vi "GOOPUtil_GetClassMembers.vi"(0 "LVClassPath":path, 5 "error in (no error)":errorcluster) -> (14 "MemberPaths":T1[](array[typedef]), 19 "error out":errorcluster)   [LabVIEW 2012, in "GOOPUtility.lvlib"]
doc: "Returns all class members paths, names and scopes (except the util VIs) from a given GOOP class path.\n\nNote: This will not work if the .lvclass file is inside an .exe file.\n\nThis is a collection of generic GOOP utility VIs. Please notice that it is important that the frontpanel of the Create, Destroy and GetObjectStatus is not removed when building an application."
uses:
  <vilib>/addons/GOOPUtility/GOOPUtility.lvlib
  <vilib>/addons/GOOPUtility/GOOPUtil_MemberDefinition.ctl
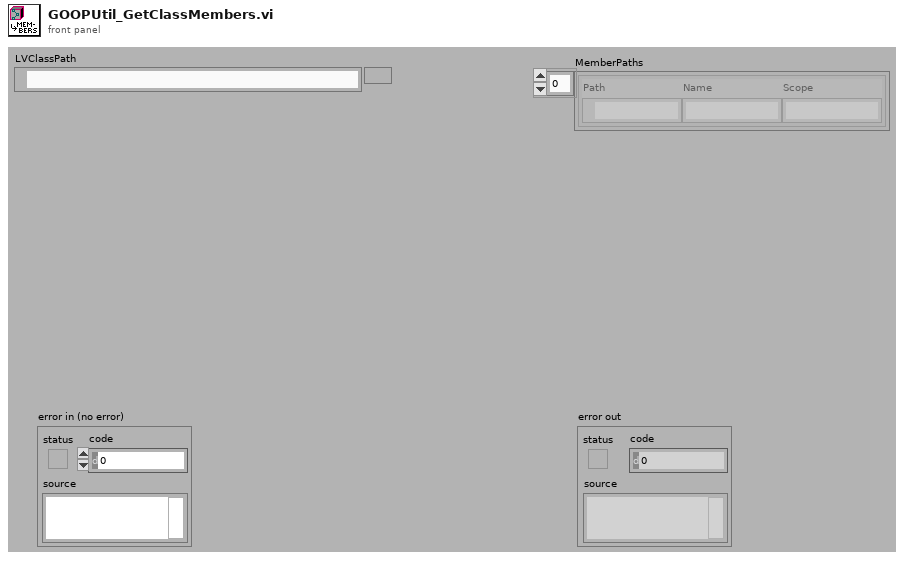
[diagram p1: front panel]
types:
  T1 = typedef "GOOPUtility.lvlib/GOOPUtil_MemberDefinition.ctl" = cluster{"Path":path, "Name":string, "Scope":string}
  T2 = enum16{"open", "replace", "create", "open or create", "replace or create", "replace or create with confirmation"}
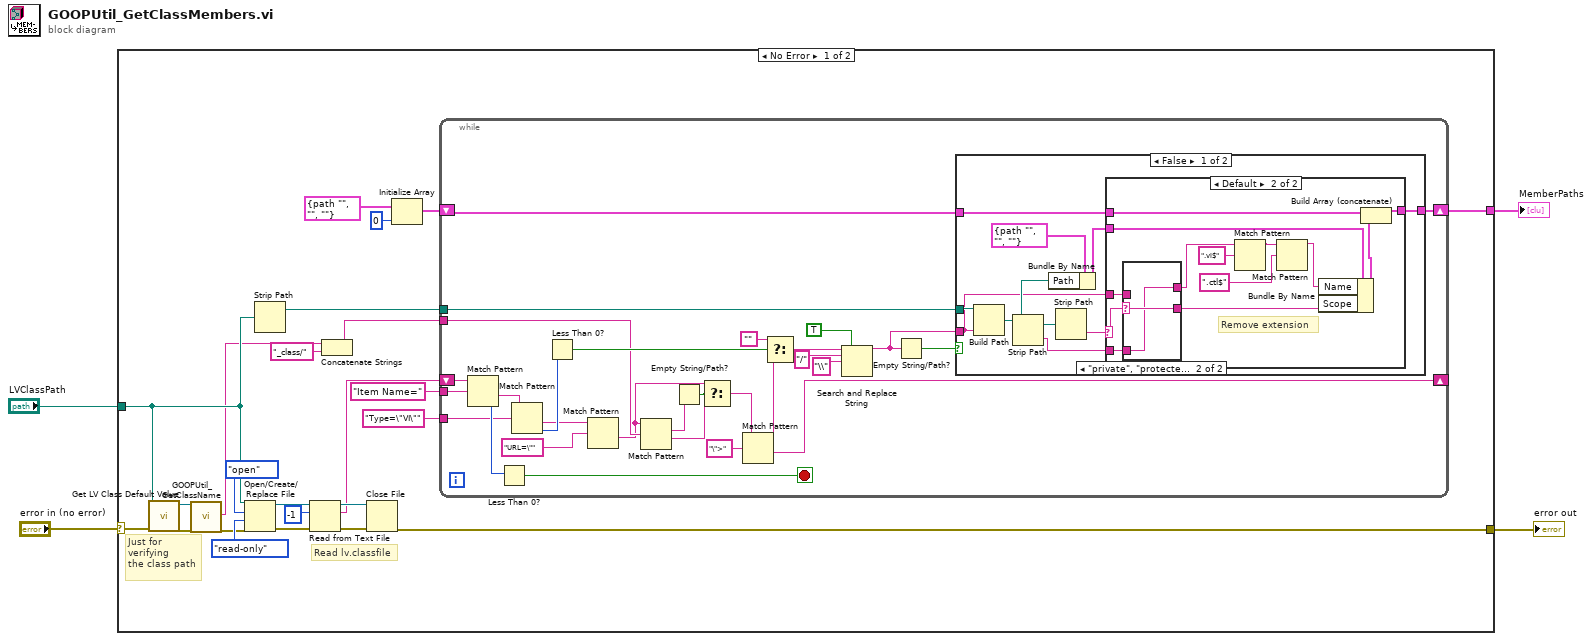
[diagram p0: block diagram]
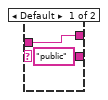
[diagram p3: hidden frame]
diagram:
  n1 = case shown="No Error" "error in (no error)" {
    selector: "error in (no error)" -> [w17 w87]
    tunnel: [w19 w87] -> w3
    tunnel: "LVClassPath" -> [w16 _]
    tunnel: [w14 _] -> w1
    frame No Error {
      # "Read lv.classfile"
      # "Just for\nverifying\nthe class path"
      n2 = call <vilib>:"Get LV Class Default Value.vi"("error in (no error)"=w17, "class path"=w16) -> ("error out"=w10:errorcluster, "object"=w9:refnum<class>)  [unwired: 8 in]
      n3 = call <vilib>:"GOOPUtil_GetClassName.vi"("LabVIEW Object"=w9, "error in (no error)"=w10) -> ("Class Name"=w7:string, "error out"=w8:errorcluster)  [unwired: 13 in, 3 out]
      n4 = Open/Create/Replace File(file path (use dialog)=w16, error in=w8, operation (0:open)=T2."open", access (0:read/write)=enum16{"read/write", "read-only", "write-only"}."read-only") -> (refnum out=w27:refnum<file>, error out=w26:errorcluster)  [unwired: 2 in, 1 out]
      n5 = Strip Path(path=w16) -> (stripped path=w15:path)  [unwired: 1 out]
      n6 = Read from Text File(file (use dialog)=w27, count=-1, error in=w26) -> (refnum out=w23:refnum<file>, text=w20:string, error out=w24:errorcluster)  [unwired: 2 out]
      n7 = Concatenate Strings(w7, "_class/" ("string")) -> (w5:string)
      n8 = Close File(refnum=w23, error in=w24) -> (error out=w19:errorcluster)  [unwired: 1 out]
      n9 = Initialize Array(T1 {"Path"=path "", "Name"="", "Scope"=""} ("Member"), 0 ("dimension size")) -> (w13:T1[])
      n10 = while {
        shift-right: [w44] -> _
        shift-left: w20 -> [w57]
        tunnel: "Item Name=" ("Search Tag") -> [w53]
        tunnel: "Type=\"VI\"" ("regular expression") -> [w52]
        shift-right: [w35] -> w14
        shift-left: w13 -> [w38]
        tunnel: w15 -> [w37]
        tunnel: w5 -> [w34]
        stop <- w54 stop-if-true
        n11 = Match Pattern(string=w57, regular expression=w53) -> (after substring=w56:string, offset past match=w55:i32)  [unwired: 3 out]
        n12 = Less Than 0?(x=w55) -> (x < 0?=w54:bool)
        n13 = Match Pattern(string=w56, regular expression=w52) -> (after substring=w48:string, offset past match=w51:i32)  [unwired: 3 out]
        n14 = Less Than 0?(x=w51) -> (x < 0?=w49:bool)
        n15 = Match Pattern(string=w48, regular expression="URL=\"" ("search string/char (-)")) -> (after substring=w31:string)  [unwired: 4 out]
        n16 = Match Pattern(string=w31, regular expression=w34) -> (match substring=w33:string, after substring=w30:string)  [unwired: 3 out]
        n17 = Empty String/Path?(string/path=w33) -> (empty?=w32:bool)
        n18 = Select(t=w31, s=w32, f=w30) -> (s? t:f=w29:string)
        n19 = Match Pattern(string=w29, regular expression="\">" ("search string/char (-)")) -> (before substring=w45:string, after substring=w44:string)  [unwired: 3 out]
        n20 = Select(t="", s=w49, f=w45) -> (s? t:f=w43:string)
        n21 = Search and Replace String(replace all?=TRUE ("replace all? (F)"), input string=w43, search string="/" ("search string/char (-)"), replace string="\\" ("search string/char (-)")) -> (result string=w36:string)  [unwired: 1 in, 6 out]
        n22 = Empty String/Path?(string/path=w36) -> (empty?=w39:bool)
        n23 = case shown="False" w39 {
          tunnel: w38 -> [w67 w86]
          tunnel: w37 -> [w66 _]
          tunnel: w36 -> [w59 _]
          tunnel: [w65 w86] -> w35
          frame False {
            n24 = Build Path(base path=w66, name or relative path=w59) -> (appended path=w61:path)
            n25 = Strip Path(path=w61) -> (stripped path=w64:path, name=w58:string)
            n26 = Bundle By Name(cluster=T1 {"Path"=path "", "Name"="", "Scope"=""} ("Member"), "Path"=w61) -> (w60:T1)
            n27 = Strip Path(path=w64) -> (name=w63:string)  [unwired: 1 out]
            n28 = case shown="Default" w63 {
              selector: w63 -> [_ w77]
              tunnel: w67 -> [w68 w81]
              tunnel: [w68 w78] -> w65
              tunnel: w60 -> [_ w80]
              tunnel: w59 -> [_ w75]
              tunnel: w58 -> [_ w74]
              frame "utils" {
                # "Don't include the utils VIs that is only for\nthe GOOP implementation."
              }
              frame Default {
                # "Remove extension"
                n29 = case shown="\"private\", \"protected\"" w77 {
                  selector: w77 -> [_ w85]
                  tunnel: ["public" w85] -> w76
                  tunnel: w75 -> [w82 _]
                  tunnel: w74 -> [_ w84]
                  tunnel: [w82 w84] -> w72
                  frame Default {
                  }
                  frame "private", "protected" {
                  }
                }
                n30 = Match Pattern(string=w72, regular expression=".vi$") -> (before substring=w71:string)  [unwired: 1 in, 3 out]
                n31 = Match Pattern(string=w71, regular expression=".ctl$") -> (before substring=w70:string)  [unwired: 1 in, 3 out]
                n32 = Bundle By Name(cluster=w80, "Name"=w70, "Scope"=w76) -> (w79:T1)
                n33 = Build Array (concatenate)(w81, w79) -> (w78:T1[])
              }
            }
          }
          frame True {
            # "False alarm..."
          }
        }
      }
    }
    frame Error {
    }
  }
  "error out" <- w3
  "MemberPaths" <- w1
